vi "Read Configuration File.vi"(8 "error in (no error)":errorcluster, 11 "Instrument in":refnum<class "Instrument.lvclass">) -> (0 "error out":errorcluster, 3 "Instrument out":refnum<class "Instrument.lvclass">)   [LabVIEW 2019, in "Instrument.lvclass"]
uses:
  Instrument.lvclass
  Instrument.lvclass/Instrument.ctl
  Configuration/Configuration.lvclass
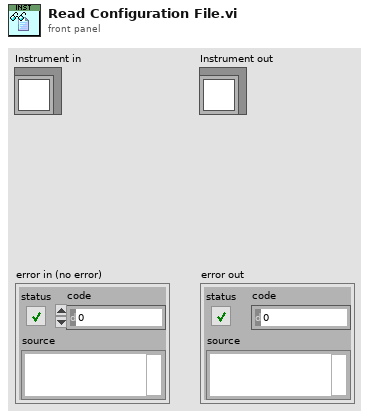
[diagram p1: front panel]
types:
  T1 = typedef "Instrument.lvclass/Configuration--Cluster.ctl" = cluster{"Hardware":T2, "SMO":T3}
  T2 = typedef "Instrument.lvclass/HW Configuration--Cluster.ctl" = cluster{"Address":string, "Type":string, "COM Type":string}
  T3 = typedef "Instrument.lvclass/SMO Configuration--Cluster.ctl" = cluster{"Address":string, "Port":u16, "RC Type":T4, "Debug Mode?":bool}
  T4 = typedef "RemoteControl.lvclass/RC Com Type--enum.ctl" = enum16{"RC", "STM", "ZMQ"}
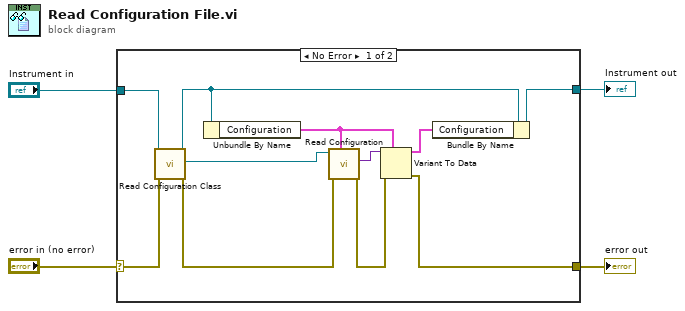
[diagram p0: block diagram]
diagram:
  n1 = case shown="No Error" "error in (no error)" {
    selector: "error in (no error)" -> [w5 w17]
    tunnel: [w13 w17] -> w4
    tunnel: [w8 w16] -> w3
    tunnel: "Instrument in" -> [w7 w16]
    frame No Error {
      n2 = call "Read Configuration Class.vi"("error in (no error)"=w5, "Instrument in"=w7) -> ("error out"=w11:errorcluster, "Configuration.lvclass"=w12:refnum<class "Configuration.lvclass">, "Instrument out"=w6:refnum<class "Instrument.lvclass">)  [unwired: 7 in]
      n3 = Unbundle By Name(w6) -> ("Configuration"=w10:T1)
      n4 = call "Read Configuration.vi"("INI Fomatted Cluster Type"=w10, "error in (no error)"=w11, "Configuration in"=w12) -> ("error out"=w14:errorcluster, "Configuration"=w15:variant)  [unwired: 6 in, 1 out]
      n5 = Variant To Data(error in=w14, type=w10, Variant=w15) -> (data=w9:T1, error out=w13:errorcluster)
      n6 = Bundle By Name(cluster=w6, "Configuration"=w9) -> (w8:refnum<class "Instrument.lvclass">)
    }
    frame Error {
    }
  }
  "Instrument out" <- w3
  "error out" <- w4
